vi "AcknowledgeInterruptsHW.vi"(8 "error in (no error)":errorcluster, 11 "BME_DG_System in":refnum<class "BME_DG_System.lvclass">) -> (0 "error out":errorcluster, 3 "BME_DG_System out":refnum<class "BME_DG_System.lvclass">)   [LabVIEW 2009, in "POLARIS BME DG.lvlib" / "BME_DG_System.lvclass"]
uses:
  BME_DG_System.lvclass
  BME_DG_System.lvclass/BME_DG_System.ctl
  BME_DG_Base/BME_DG_Base.lvclass
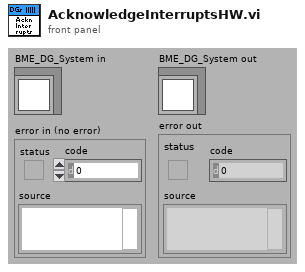
[diagram p1: front panel]
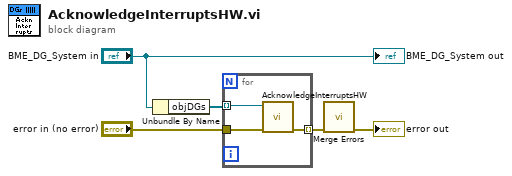
[diagram p0: block diagram]
diagram:
  n1 = Unbundle By Name("BME_DG_System in") -> ("objDGs"=w4:refnum<class "BME_DG_Base.lvclass">[])
  n2 = for {
    tunnel: w4 -> [w8] mode=indexing
    tunnel: "error in (no error)" -> [w7]
    tunnel: [w6] -> w3 mode=indexing
    n3 = call-dynamic "AcknowledgeInterruptsHW.vi"("error in (no error)"=w7, "BME_DG_Base in"=w8) -> ("error out"=w6:errorcluster)  [unwired: 8 in, 1 out]
  }
  n4 = call <vilib>:"Merge Errors.vi"("error array in"=w3) -> ("error out"=→"error out":errorcluster)  [unwired: 6 in]
  "BME_DG_System out" <- "BME_DG_System in"
